vi "get_x_fractions.vi"(8 "error in (no error)":errorcluster, 11 "TrajectoryAK101022Resonance in":refnum<class "TrajectoryAK101022Resonance.lvclass">) -> (0 "error out":errorcluster, 1 "x offset fly back fraction":dbl, 2 "x offset fly forward fraction":dbl, 3 "TrajectoryAK101022Resonance out":refnum<class "TrajectoryAK101022Resonance.lvclass">, 4 "x scan segment fraction":dbl)   [LabVIEW 2010, in "TrajectoryAK101022Resonance.lvclass"]
uses:
  TrajectoryAK101022Resonance.lvclass
  TrajectoryAK101022Resonance.lvclass/TrajectoryAK101022Resonance.ctl
  class_data.vi
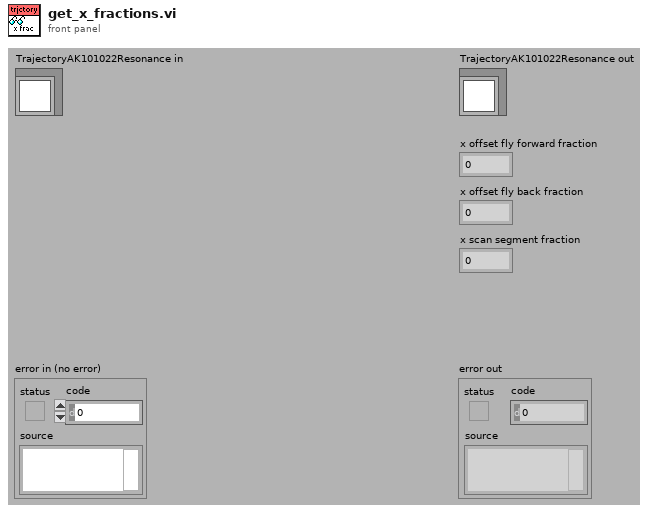
[diagram p1: front panel]
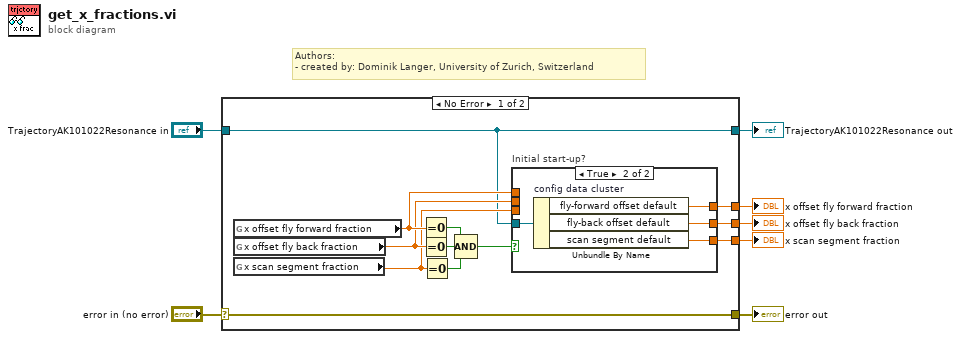
[diagram p0: block diagram]
diagram:
  # "Authors: \n- created by: Dominik Langer, University of Zurich, Switzerland"
  n1 = case shown="No Error" "error in (no error)" {
    selector: "error in (no error)" -> [w19 w28]
    tunnel: [w19 w28] -> w6
    tunnel: [w8 w27] -> w4
    tunnel: "TrajectoryAK101022Resonance in" -> [w8 w27]
    tunnel: [w15 _] -> w2
    tunnel: [w14 _] -> w3
    tunnel: [w13 _] -> w1
    frame No Error {
      n2 = global read "class_data.vi" "x offset fly forward fraction"() -> (w11:dbl)
      n3 = global read "class_data.vi" "x offset fly back fraction"() -> (w10:dbl)
      n4 = global read "class_data.vi" "x scan segment fraction"() -> (w9:dbl)
      n5 = Equal To 0?(x=w11) -> (x = 0?=w18:bool)
      n6 = Equal To 0?(x=w10) -> (x = 0?=w17:bool)
      n7 = Equal To 0?(x=w9) -> (x = 0?=w16:bool)
      n8 = Compound Arithmetic op=AND(w18, w17, w16) -> (w12:bool)
      n9 = case "Initial start-up?" shown="True" w12 {
        tunnel: w8 -> [_ w26]
        tunnel: [w22 w25] -> w15
        tunnel: [w20 w24] -> w14
        tunnel: [w21 w23] -> w13
        tunnel: w11 -> [w22 _]
        tunnel: w10 -> [w20 _]
        tunnel: w9 -> [w21 _]
        frame False {
        }
        frame True {
          n10 = Unbundle By Name "config data cluster"(w26) -> ("fly-forward offset default"=w25:dbl, "fly-back offset default"=w24:dbl, "scan segment default"=w23:dbl)
        }
      }
    }
    frame Error {
    }
  }
  "error out" <- w6
  "TrajectoryAK101022Resonance out" <- w4
  "x offset fly forward fraction" <- w2
  "x offset fly back fraction" <- w3
  "x scan segment fraction" <- w1
